vi "New Session SetUp.vi"(8 "error in (no error)":errorcluster, 10 "Stop Refnum":refnum<vi>, 11 "Generic Data Acquisition in":refnum<class "Generic Data Acquisition.lvclass">) -> (0 "error out":errorcluster, 3 "output cluster":refnum<class "Generic Data Acquisition.lvclass">)   [LabVIEW 2014, in "Generic Data Acquisition.lvlib" / "Generic Data Acquisition.lvclass"]
uses:
  Generic Data Acquisition.lvclass
  Abstract Sensor/Abstract Sensor.lvclass
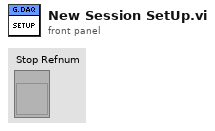
[diagram p1: front panel]
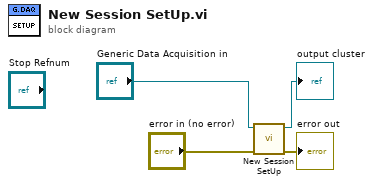
[diagram p0: block diagram]
diagram:
  n1 = call-parent "New Session SetUp.vi"("error in (no error)"="error in (no error)", "Abstract Sensor in"="Generic Data Acquisition in") -> ("error out"=→"error out":errorcluster, "Abstract Sensor out"=→"output cluster":refnum<class "Generic Data Acquisition.lvclass">)  [unwired: 8 in]
